vi "DetectedPelletPage.vi"() -> ()   [LabVIEW 2019, in "detectedPellet.lvlib"]
uses:
  detectedPellet.lvlib
panel:
  out "Number of Pellets Disc 30":u32 caption="Number of Pellets"
  out "Number of Pellets Disc 29":u32 caption="Number of Pellets"
  out "Number of Pellets Disc 28":u32 caption="Number of Pellets"
  out "Number of Pellets Disc 27":u32 caption="Number of Pellets"
  out "Number of Pellets Disc 26":u32 caption="Number of Pellets"
  out "error out":errorcluster
  in  "Close":bool
  out "Disc 30":T1(plugin-control)
  out "Disc 29":T1(plugin-control)
  out "Disc 28":T1(plugin-control)
  out "Disc 27":T1(plugin-control)
  out "Disc 26":T1(plugin-control)
  # "DSGS"
  # "Detected Pellets"
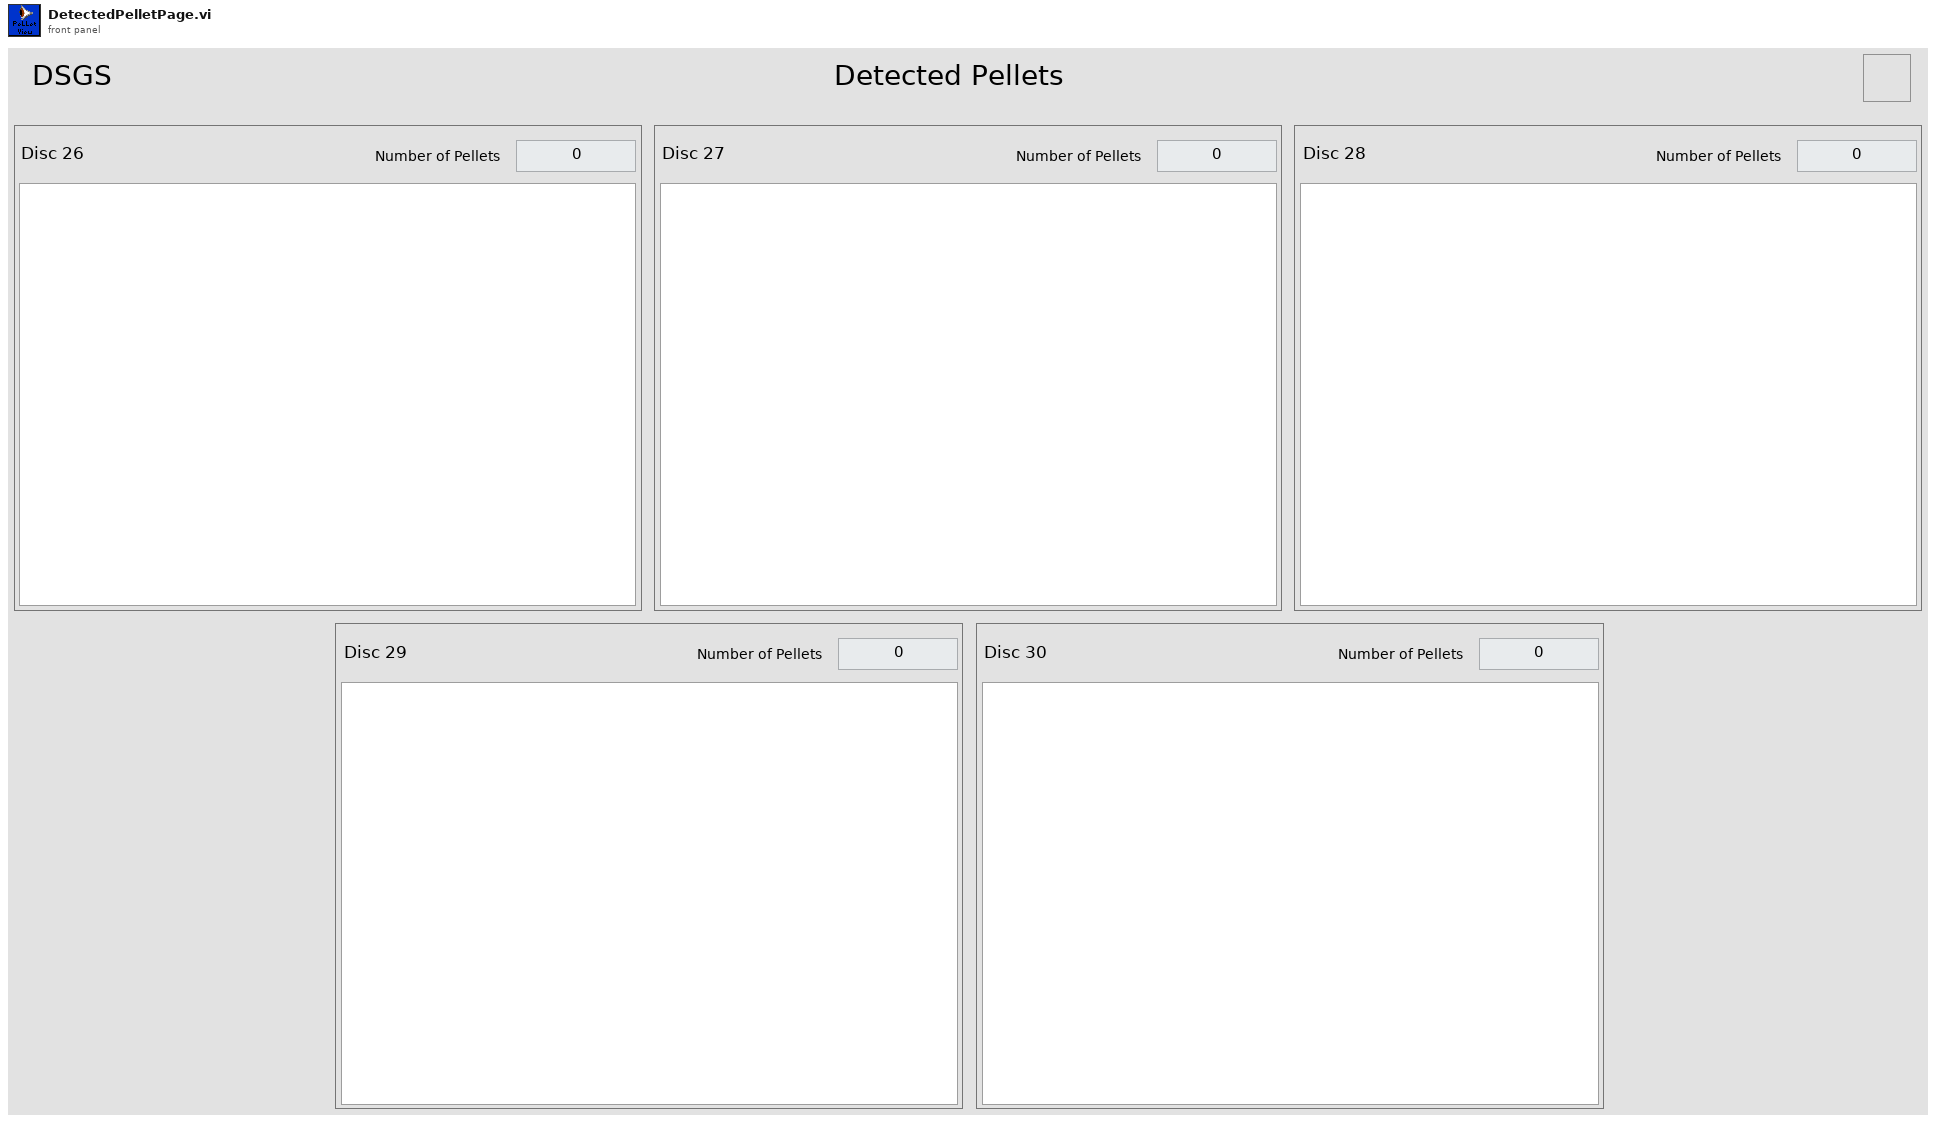
[diagram p1: front panel]
types:
  T1 = typedef "IMAQ Image.ctl" = refnum<image>
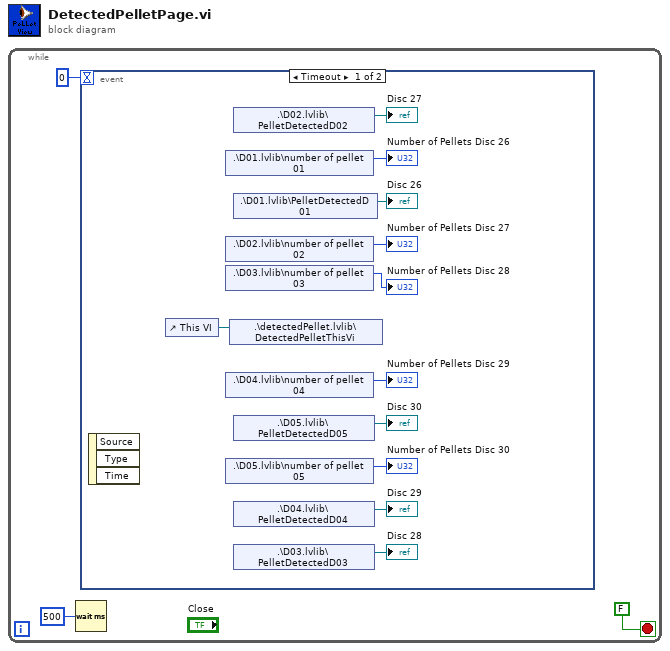
[diagram p0: block diagram]
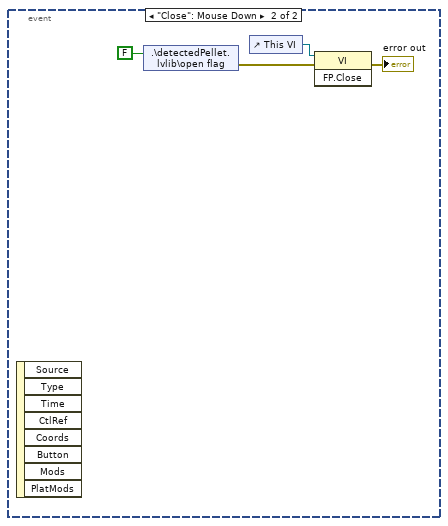
[diagram p2: hidden frame]
diagram:
  n1 = while {
    stop <- FALSE stop-if-true
    n2 = Wait (ms)(milliseconds to wait=u32 500) -> ()  [unwired: 1 out]
    n3 = event shown="[0] Timeout" {
      selector: _ -> [_ _]
      dyn-events: _ -> [_ _]
      timeout: 0 -> [_ _]
      event Timeout {
        n4 = event-data() -> ()  [unwired: 1 in, 3 out]
        n5 = control-ref of="This VI"() -> (w14:refnum<vi>)
        n6 = shared-variable ".\\D01.lvlib\\number of pellet 01"() -> (→"Number of Pellets Disc 26":u32)  [unwired: 1 in, 1 out]
        n7 = shared-variable ".\\D02.lvlib\\number of pellet 02"() -> (→"Number of Pellets Disc 27":u32)  [unwired: 1 in, 1 out]
        n8 = shared-variable ".\\D03.lvlib\\number of pellet 03"() -> (→"Number of Pellets Disc 28":u32)  [unwired: 1 in, 1 out]
        n9 = shared-variable ".\\D04.lvlib\\number of pellet 04"() -> (→"Number of Pellets Disc 29":u32)  [unwired: 1 in, 1 out]
        n10 = shared-variable ".\\D05.lvlib\\number of pellet 05"() -> (→"Number of Pellets Disc 30":u32)  [unwired: 1 in, 1 out]
        n11 = shared-variable ".\\detectedPellet.lvlib\\DetectedPelletThisVi"(w14) -> ()  [unwired: 1 in, 1 out]
        n12 = shared-variable ".\\D02.lvlib\\PelletDetectedD02"() -> (→"Disc 27":refnum<image>)  [unwired: 1 in, 1 out]
        n13 = shared-variable ".\\D01.lvlib\\PelletDetectedD 01"() -> (→"Disc 26":refnum<image>)  [unwired: 1 in, 1 out]
        n14 = shared-variable ".\\D05.lvlib\\PelletDetectedD05"() -> (→"Disc 30":refnum<image>)  [unwired: 1 in, 1 out]
        n15 = shared-variable ".\\D04.lvlib\\PelletDetectedD04"() -> (→"Disc 29":refnum<image>)  [unwired: 1 in, 1 out]
        n16 = shared-variable ".\\D03.lvlib\\PelletDetectedD03"() -> (→"Disc 28":refnum<image>)  [unwired: 1 in, 1 out]
      }
      event "Close": Mouse Down {
        n17 = event-data() -> ()  [unwired: 1 in, 8 out]
        n18 = shared-variable ".\\detectedPellet.lvlib\\open flag"(FALSE ("open flag")) -> (error out=w16:errorcluster)  [unwired: 1 in]
        n19 = control-ref of="This VI"() -> (w18:refnum<vi>)
        n20 = invoke class="VI" method="FP.Close"(reference=w18, error in=w16) -> (error out=→"error out":errorcluster)  [unwired: 1 in, 2 out]
      }
    }
  }
